vi "Query Amplitude.vi"(8 "error in (no error)":errorcluster, 11 "VISA resource name":refnum<visa-resource-name>) -> (0 "error out":errorcluster, 2 "Amplitude (dBm)":dbl, 3 "VISA resource name out":refnum<visa-resource-name>)   [LabVIEW 2009, in "Agilent PSG MXG Series.lvlib"]
uses:
  Agilent PSG MXG Series.lvlib
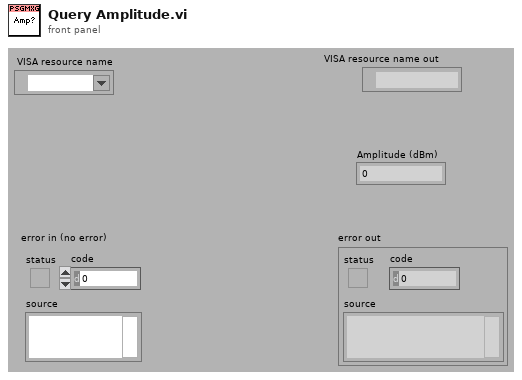
[diagram p1: front panel]
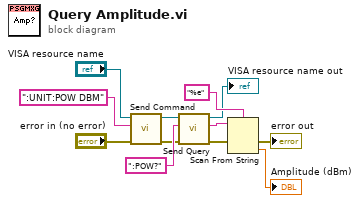
[diagram p0: block diagram]
diagram:
  n1 = call "Send Command.vi"("error in (no error)"="error in (no error)", "write buffer"=":UNIT:POW DBM", "VISA resource name"="VISA resource name") -> ("error out"=w4:errorcluster, "VISA resource name out"=w6:refnum<visa-resource-name>)  [unwired: 7 out]
  n2 = call "Send Query.vi"("error in (no error)"=w4, "write buffer"=":POW?", "VISA resource name"=w6) -> ("error out"=w2:errorcluster, "read buffer"=w11:string, "VISA resource name out"=→"VISA resource name out":refnum<visa-resource-name>)  [unwired: 6 out]
  n3 = Scan From String(format string="%e", input string=w11, error in=w2) -> (error out=→"error out":errorcluster, output 1=→"Amplitude (dBm)":dbl)  [unwired: 1 in, 3 out]
